vi "parse -- find first line.vi"(7 "regexp":string="(\\s*[\\d\\.\\+\\-]+)+\\s*\\r?", 11 "string array":string[](array[string])=["eee d", "4", "12 34.0 56", "1 23 4", "yy uu iii oo"]) -> (0 "line and after":string[](array[string])=["12 34.0 56", "1 23 4", "yy uu iii oo"], 1 "before":string[](array[string])=["eee d"], 2 "matching line":string="4", 3 "after":string[](array[string])=["12 34.0 56", "1 23 4", "yy uu iii oo"], 4 "index":i32)   [LabVIEW 2015]
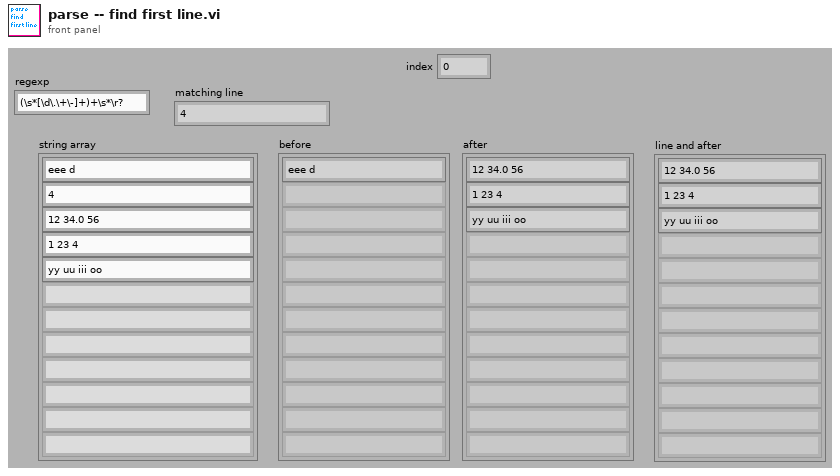
[diagram p1: front panel]
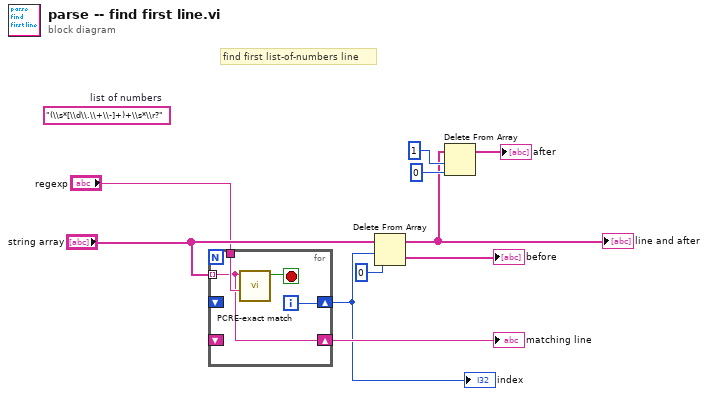
[diagram p0: block diagram]
diagram:
  (unwired) "(\\s*[\\d\\.\\+\\-]+)+\\s*\\r?"  # list of numbers
  # "find first list-of-numbers line"
  n1 = for {
    tunnel: "string array" -> [w11] mode=indexing
    shift-right: [w13] -> w5
    shift-left: _ -> [_]
    tunnel: "regexp" -> [w12]
    shift-right: [w11] -> w7
    shift-left: _ -> [_]
    i -> [w13]
    stop <- w14 stop-if-true
    n2 = call "PCRE-exact match.vi"("regular expression"=w12, "input string"=w11) -> ("exact match"=w14:bool)  [unwired: 7 in, 2 out]
  }
  "matching line" <- w7
  "index" <- w5
  n3 = Delete From Array(array="string array", length=w5, index=0 ("index (row)")) -> (deleted portion=→"before":string[], array with subset deleted=w1:string[])
  "line and after" <- w1
  n4 = Delete From Array(array=w1, length=1 ("index (row)"), index=0 ("index (row)")) -> (array with subset deleted=→"after":string[])  [unwired: 1 out]
